vi "Get Table Column Range.vi"(7 "Sheet Name in":string, 8 "error in":errorcluster, 9 "Column Name":string, 10 "Table Name":string, 11 "SpreadsheetDoc in":refnum<k24>) -> (0 "error out":errorcluster, 1 "Row Count":i32, 2 "Range":string, 3 "SpreadsheetDoc out":refnum<k24>, 5 "Sheet Name out":string)   [LabVIEW 2019, in "Open Xml.lvlib"]
uses:
  Open Xml.lvlib
  D:/git/Open-Xml-LabVIEW/Source/DocumentFormat.OpenXml.dll
  DocumentFormat.OpenXml.dll
  D:/git/Open-Xml-LabVIEW/Source/DocumentFormat.OpenXml.Framework.dll
  DocumentFormat.OpenXml.Framework.dll
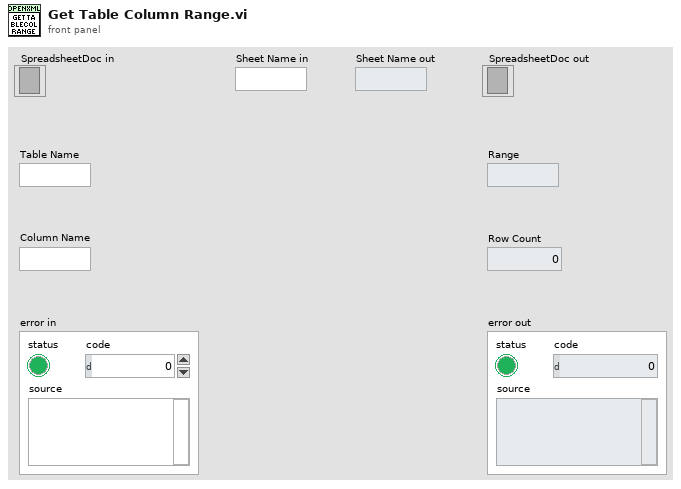
[diagram p1: front panel]
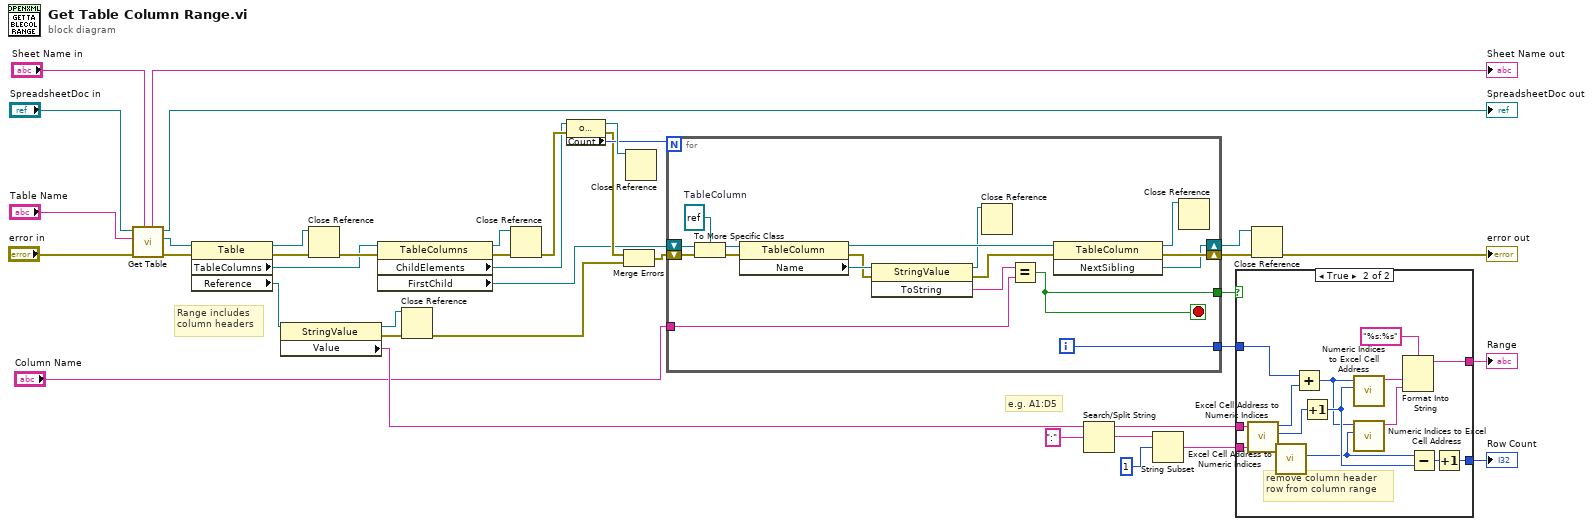
[diagram p0: block diagram]
diagram:
  # "e.g. A1:D5"
  # "Range includes\ncolumn headers"
  n1 = call "Get Table.vi"("Sheet Name in"="Sheet Name in", "error in"="error in", "Table Name"="Table Name", "SpreadsheetDoc in"="SpreadsheetDoc in") -> ("error out"=w9:errorcluster, "Table"=w8:refnum<k24>, "SpreadsheetDoc out"=→"SpreadsheetDoc out":refnum<k24>, "Sheet Name out"=→"Sheet Name out":string)  [unwired: 4 in]
  n2 = property class="Table"(reference=w8, error in=w9) -> (reference out=w17:refnum<k24>, error out=w14:errorcluster, "TableColumns"=w15:refnum<k24>, "Reference"=w28:refnum<k24>)
  n3 = property class="StringValue"(reference=w28) -> (reference out=w30:refnum<k24>, error out=w29:errorcluster, "Value"=w31:string)  [unwired: 1 in]
  n4 = Close Reference(reference=w17, error in (no error)=w14) -> (error out=w16:errorcluster)
  n5 = property class="TableColumns"(reference=w15, error in=w16) -> (reference out=w22:refnum<k24>, error out=w11:errorcluster, "ChildElements"=w19:refnum<k24>, "FirstChild"=w13:refnum<k24>)
  n6 = Close Reference(reference=w30, error in (no error)=w29) -> (error out=w25:errorcluster)
  n7 = Close Reference(reference=w22, error in (no error)=w11) -> (error out=w21:errorcluster)
  n8 = property class="OpenXmlElementList"(reference=w19, error in=w21) -> (reference out=w23:refnum<k24>, error out=w18:errorcluster, "Count"=w20:i32)
  n9 = Merge Errors(w18, w25) -> (w24:errorcluster)
  n10 = Close Reference(reference=w23) -> ()  [unwired: 1 in, 1 out]
  n11 = for {
    N: w20 -> [_]
    shift-right: [w50] -> w12
    shift-left: w24 -> [w53]
    tunnel: "Column Name" -> [w46]
    shift-right: [w48] -> w27
    shift-left: w13 -> [w55]
    tunnel: [w47] -> w34
    tunnel: [w40] -> w1
    i -> [w47]
    stop <- w40 stop-if-true
    w54 = refnum<k24> refnum  # TableColumn
    n12 = To More Specific Class(target class=w54, reference=w55, error in=w53) -> (specific class reference=w52:refnum<k24>, error out=w56:errorcluster)
    n13 = property class="TableColumn"(reference=w52, error in=w56) -> (reference out=w49:refnum<k24>, error out=w45:errorcluster, "Name"=w51:refnum<k24>)
    n14 = invoke class="StringValue" method="ToString"(reference=w51, error in=w45) -> (reference out=w43:refnum<k24>, error out=w44:errorcluster, "ToString"=w42:string)  [unwired: 1 in]
    n15 = Close Reference(reference=w43) -> ()  [unwired: 1 in, 1 out]
    n16 = Equal?(x=w42, y=w46) -> (x = y?=w40:bool)
    n17 = invoke class="TableColumn" method="NextSibling"(reference=w49, error in=w44) -> (reference out=w41:refnum<k24>, error out=w50:errorcluster, "NextSibling"=w48:refnum<k24>)  [unwired: 1 in]
    n18 = Close Reference(reference=w41) -> ()  [unwired: 1 in, 1 out]
  }
  n19 = Search/Split String(string=w31, search string/char (-)=":" ("Split Pattern")) -> (substring before match=w33:string, match + rest of string=w35:string)  [unwired: 1 in, 1 out]
  n20 = String Subset(string=w35, offset (0)=1) -> (substring=w37:string)  [unwired: 1 in]
  n21 = case shown="True" w1 {
    tunnel: [_ w57] -> w39
    tunnel: [_ w67] -> w38
    tunnel: w37 -> [_ w64]
    tunnel: w34 -> [_ w59]
    tunnel: w33 -> [_ w58]
    frame False {
    }
    frame True {
      # "remove column header\nrow from column range"
      n22 = call "Excel Cell Address to Numeric Indices.vi"("Cell Name"=w58) -> ("Row Number"=w61:i32, "Column Number"=w60:i32)  [unwired: 9 in]
      n23 = call "Excel Cell Address to Numeric Indices.vi"("Cell Name"=w64) -> ("Row Number"=w68:i32)  [unwired: 9 in, 1 out]
      n24 = Add(x=w59, y=w60) -> (x+y=w65:i32)
      n25 = Increment(x=w61) -> (x+1=w69:i32)
      n26 = call "Numeric Indices to Excel Cell Address.vi"("Row"=w69, "Column"=w65) -> ("Cell Address"=w63:string)  [unwired: 9 in]
      n27 = call "Numeric Indices to Excel Cell Address.vi"("Row"=w68, "Column"=w65) -> ("Cell Address"=w66:string)  [unwired: 9 in]
      n28 = Format Into String(format string="%s:%s", w63, w66) -> (resulting string=w67:string)  [unwired: 2 in, 1 out]
      n29 = Subtract(x=w68, y=w69) -> (x-y=w70:i32)
      n30 = Increment(x=w70) -> (x+1=w57:i32)
    }
  }
  "Row Count" <- w39
  "Range" <- w38
  n31 = Close Reference(reference=w27, error in (no error)=w12) -> (error out=→"error out":errorcluster)
